vi "Build Channel Settings.vi"(8 "error in":errorcluster, 11 "Node Ptr":T1 format="%.0x") -> (0 "error out":errorcluster, 2 "Channel Settings Table":string[][](array[string]), 3 "Node Ptr out":T1=18446744073709551615 format="%.0x")   [LabVIEW 2026, in "SystemMonitor System Explorer.lvlib"]
uses:
  SystemMonitor System Explorer.lvlib
  <vilib>/NI VeriStand/Custom Device API/Custom Device Item Ref.ctl
  <vilib>/NI VeriStand/Custom Device API/Custom Device API.lvlib
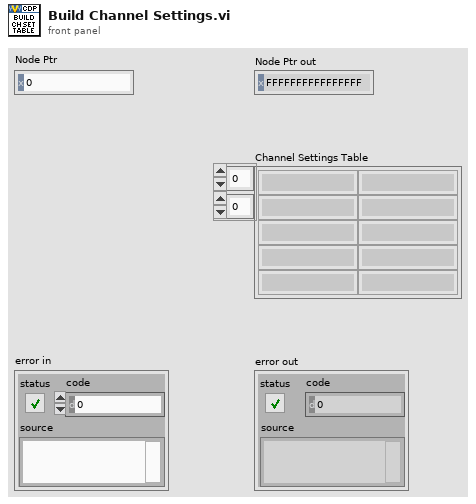
[diagram p1: front panel]
types:
  T1 = typedef "Custom Device API.lvlib/Custom Device Item Ref.ctl" = u64
  T2 = typedef "Custom Device API.lvlib/Custom Device Channel.ctl" = cluster{"Type":T3, "Units":string, "Default Value":dbl, "Faultable":bool, "Scalable":bool}
  T3 = typedef "Custom Device API.lvlib/Custom Device Channel Type.ctl" = enum16{"Input", "Output"}
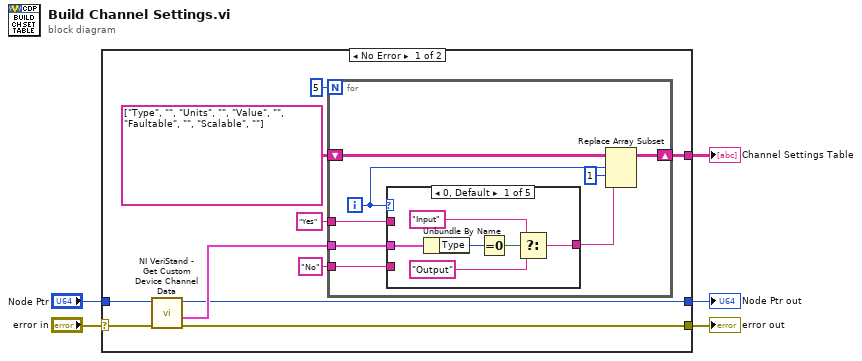
[diagram p0: block diagram]
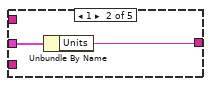
[diagram p2: hidden frame]
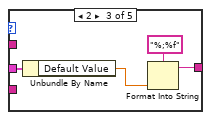
[diagram p3: hidden frame]
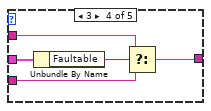
[diagram p4: hidden frame]
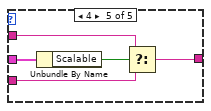
[diagram p5: hidden frame]
diagram:
  n1 = case shown="No Error" "error in" {
    selector: "error in" -> [w10 w47]
    tunnel: [w11 _] -> w5
    tunnel: [w9 w47] -> w3
    tunnel: "Node Ptr" -> [w8 w46]
    tunnel: [w6 w46] -> w1
    frame No Error {
      n2 = call <vilib>:"NI VeriStand - Get Custom Device Channel Data.vi"("error in (no error)"=w10, "Channel Ref in"=w8) -> ("error out"=w9:errorcluster, "Channel"=w7:T2, "Channel Ref out"=w6:T1)  [unwired: 4 in, 3 out]
      n3 = for {
        N: 5 -> [_]
        tunnel: w7 -> [w23]
        shift-right: [w21] -> w11
        shift-left: string[][] [["Type", ""], ["Units", ""], ["Value", ""], ["Faultable", ""], ["Scalable", ""]] -> [w22]
        tunnel: "Yes" -> [w20]
        tunnel: "No" -> [w19]
        i -> [w17]
        n4 = case shown="0, Default" w17 {
          tunnel: w23 -> [w29 w31 w35 w40 w45]
          tunnel: w20 -> [_ _ _ w37 w42]
          tunnel: w19 -> [_ _ _ w38 w43]
          tunnel: [w28 w30 w32 w36 w41] -> w18
          frame 0, Default {
            n5 = Unbundle By Name(w29) -> ("Type"=w25:T3)
            n6 = Equal To 0?(x=w25) -> (x = 0?=w24:bool)
            n7 = Select(t="Input", s=w24, f="Output") -> (s? t:f=w28:string)
          }
          frame 1 {
            n8 = Unbundle By Name(w31) -> ("Units"=w30:string)
          }
          frame 2 {
            n9 = Unbundle By Name(w35) -> ("Default Value"=w33:dbl)
            n10 = Format Into String(format string="%;%f", w33) -> (resulting string=w32:string)  [unwired: 2 in, 1 out]
          }
          frame 3 {
            n11 = Unbundle By Name(w40) -> ("Faultable"=w39:bool)
            n12 = Select(t=w37, s=w39, f=w38) -> (s? t:f=w36:string)
          }
          frame 4 {
            n13 = Unbundle By Name(w45) -> ("Scalable"=w44:bool)
            n14 = Select(t=w42, s=w44, f=w43) -> (s? t:f=w41:string)
          }
        }
        n15 = Replace Array Subset(array=w22, new element=w18, index (row)=w17, index (col)=1 ("disabled index (col)")) -> (w21:string[][])
      }
    }
    frame Error {
    }
  }
  "Channel Settings Table" <- w5
  "error out" <- w3
  "Node Ptr out" <- w1
